vi "CC Parse Declination.vi"(8 "error in (no error)":errorcluster, 11 "Declination string":string) -> (0 "error out":errorcluster, 2 "Angle":dbl, 3 "Declination":T1={"Degrees"=0.0, "Arc Min"=0.0, "Arc Sec"=0.0, "Sign"=1.0})   [LabVIEW 2024]
uses:
  Telescope/Telescope cluster Declination.ctl
  <vilib>/regexp/Match Regular Expression.xnode
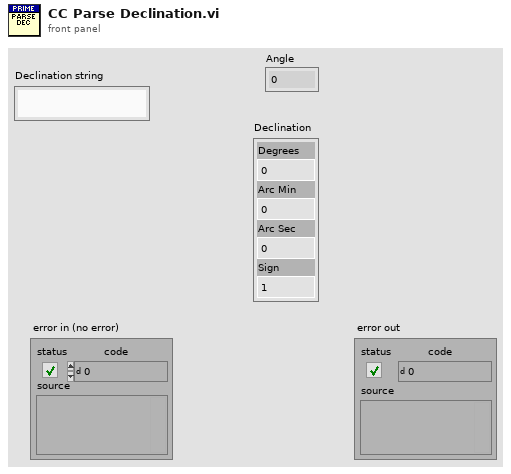
[diagram p1: front panel]
types:
  T1 = typedef "Telescope cluster Declination.ctl" = cluster{"Degrees":dbl, "Arc Min":dbl, "Arc Sec":dbl, "Sign":dbl}
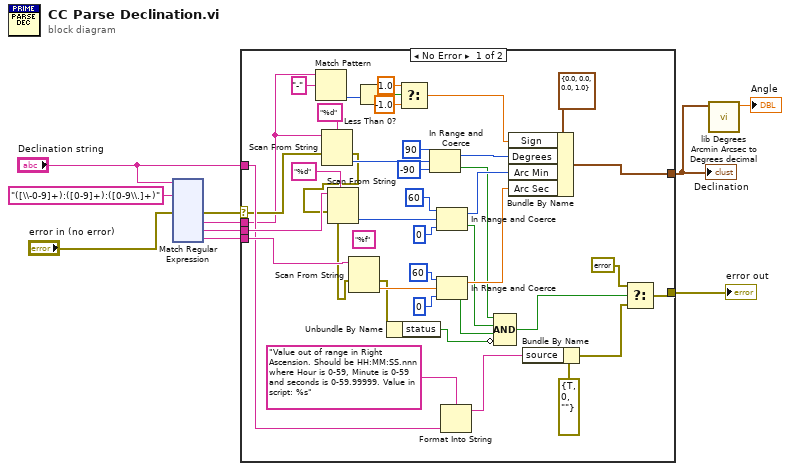
[diagram p0: block diagram]
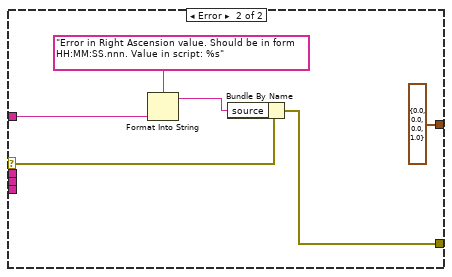
[diagram p2: hidden frame]
diagram:
  n1 = xnode "Match Regular Expression"("input string"="Declination string", "regular expression"="([\\-0-9]+):([0-9]+):([0-9\\.]+)", "error in"="error in (no error)") -> ("error out"=w5:errorcluster, "submatch 1"=w9:string, "submatch 2"=w8:string, "submatch 3"=w7:string)  [unwired: 3 in, 4 out]
  n2 = case shown="No Error" w5 {
    selector: w5 -> [w24 w55]
    tunnel: w9 -> [w17 _]
    tunnel: w8 -> [w50 _]
    tunnel: w7 -> [w49 _]
    tunnel: [w36 T1 {"Degrees"=0.0, "Arc Min"=0.0, "Arc Sec"=0.0, "Sign"=1.0} ("Declination")] -> w2
    tunnel: "Declination string" -> [w27 w56]
    tunnel: [w25 w53] -> w3
    frame No Error {
      (unwired) "%f" ("format string")
      n3 = Match Pattern(string=w17, regular expression="-") -> (offset past match=w15:i32)  [unwired: 1 in, 3 out]
      n4 = Scan From String(format string="%d", input string=w17, error in=w24) -> (error out=w23:errorcluster, output 1=w48:i32)  [unwired: 2 in, 2 out]
      n5 = Scan From String(format string="%d", input string=w50, error in=w23) -> (error out=w22:errorcluster, output 1=w45:i32)  [unwired: 2 in, 2 out]
      n6 = Scan From String(input string=w49, error in=w22) -> (error out=w21:errorcluster, output 1=w40:dbl)  [unwired: 3 in, 2 out]
      n7 = Less Than 0?(x=w15) -> (x < 0?=w14:bool)
      n8 = Unbundle By Name(w21) -> ("status"=w20:bool)
      n9 = Select(t=1.0, s=w14, f=-1.0) -> (s? t:f=w11:dbl)
      n10 = In Range and Coerce(upper limit=90, x=w48, lower limit=-90) -> (coerced(x)=w39:i32, In Range?=w35:bool)
      n11 = In Range and Coerce(upper limit=60, x=w45, lower limit=0) -> (coerced(x)=w38:i32, In Range?=w34:bool)
      n12 = In Range and Coerce(upper limit=60, x=w40, lower limit=0) -> (coerced(x)=w37:dbl, In Range?=w33:bool)
      n13 = Format Into String(format string="Value out of range in Right Ascension. Should be HH:MM:SS.nnn where Hour is 0-59, Minute is 0-59 and seconds is 0-59.99999. Value in script: %s", w27) -> (resulting string=w26:string)  [unwired: 2 in, 1 out]
      n14 = Compound Arithmetic op=AND(w35, w34, w33, invert w20) -> (w32:bool)
      n15 = Bundle By Name(cluster=T1 {"Degrees"=0.0, "Arc Min"=0.0, "Arc Sec"=0.0, "Sign"=1.0} ("Declination"), "Sign"=w11, "Degrees"=w39, "Arc Min"=w38, "Arc Sec"=w37) -> (w36:T1)
      n16 = Bundle By Name(cluster=errorcluster {"status"=TRUE, "code"=0, "source"=""} ("error out"), "source"=w26) -> (w30:errorcluster)
      n17 = Select(t=errorcluster {"status"=FALSE, "code"=0, "source"=""}, s=w32, f=w30) -> (s? t:f=w25:errorcluster)
    }
    frame Error {
      n18 = Format Into String(format string="Error in Right Ascension value. Should be in form HH:MM:SS.nnn. Value in script: %s", w56) -> (resulting string=w54:string)  [unwired: 2 in, 1 out]
      n19 = Bundle By Name(cluster=w55, "source"=w54) -> (w53:errorcluster)
    }
  }
  "error out" <- w3
  "Declination" <- w2
  n20 = call "lib Degrees Arcmin Arcsec to Degrees decimal.vi"("Declination"=w2) -> ("Angle"=→"Angle":dbl)  [unwired: 9 in, 1 out]
